vi "parseXML.vi"(8 "error in (no error)":errorcluster, 10 "XMLString in":string, 11 "Element in":refnum<class "XMLParser.lvclass">) -> (0 "error out":errorcluster, 3 "Element out":refnum<class "XMLParser.lvclass">)   [LabVIEW 2016, in "XML.lvlib" / "XMLParser.lvclass"]
doc: "The main parse VI that is called at every level in the hierarchy simply calls private methods to parse the XML."
uses:
  <userlib>/Common/XML/XMLParser/XMLParser.lvclass
  <userlib>/Common/XML/XMLParser/XMLParser.lvclass/XMLParser.ctl
  <userlib>/Common/XML/XMLParser/detElementNameNoAttributes.vi
  <userlib>/Common/XML/XMLParser/detElementNameWithAttributes.vi
  <userlib>/Common/XML/XMLParser/stripElementTags.vi
  <userlib>/Common/XML/XMLParser/replaceEmptyTagNotation.vi
  <userlib>/Common/XML/XMLAttributeParser/checkForFirstLineAttributes.vi
  <vilib>/Utility/error.llb/Trim Whitespace.vi
  <userlib>/Common/XML/XMLAttributeParser/detAttributeString.vi
  <vilib>/Utility/error.llb/Error Cluster From Error Code.vi
  <userlib>/Common/XML/XMLAttributeParser/parseAttributeData.vi
  <userlib>/Common/XML/XMLAttributeParser/removeFirstLineAttributes.vi
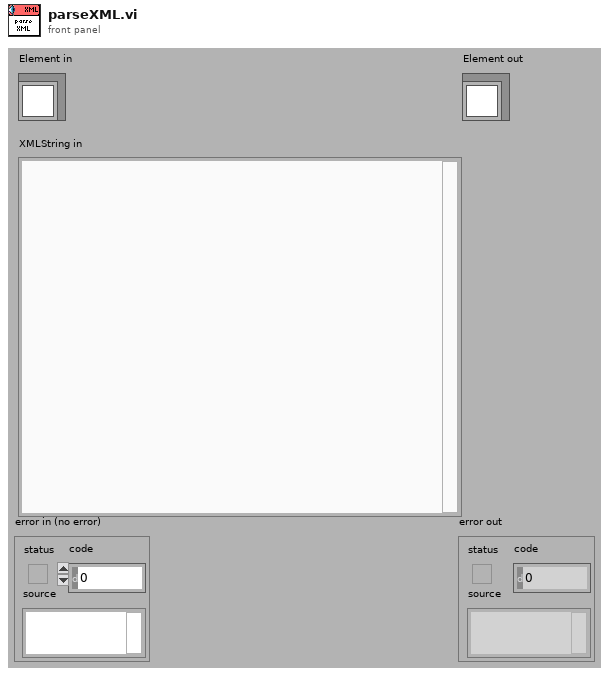
[diagram p1: front panel]
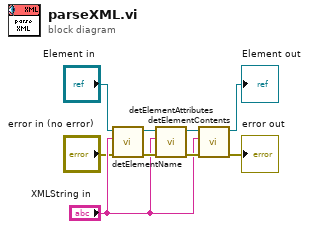
[diagram p0: block diagram]
diagram:
  n1 = call <userlib>:"detElementName.vi"("error in (no error)"="error in (no error)", "XML In"="XMLString in", "Element in"="Element in") -> ("error out"=w6:errorcluster, "Element out"=w9:refnum<class "XMLParser.lvclass">)  [unwired: 7 in]
  n2 = call <userlib>:"detElementAttributes.vi"("error in (no error)"=w6, "XMLString in"="XMLString in", "Element in"=w9) -> ("error out"=w5:errorcluster, "Element out"=w8:refnum<class "XMLParser.lvclass">)  [unwired: 7 in]
  n3 = call <userlib>:"detElementContents.vi"("error in (no error)"=w5, "XMLString in"="XMLString in", "Element in"=w8) -> ("error out"=→"error out":errorcluster, "Element out"=→"Element out":refnum<class "XMLParser.lvclass">)  [unwired: 7 in]
